vi "TEST - to Line Protocol.vi"() -> ()   [LabVIEW 2020, in "InfluxDB v2 Client.lvlib"]
doc: "Test-VI for \"to Line protocol.vi\""
uses:
  InfluxDB v2 Client.lvlib
  Tag.ctl
  Field.ctl
  Timestamp precision.ctl
  Data Point.ctl
  Data Type.ctl
panel:
  in  "Timestamp precision":T1
  in  "Use Timestamp?":bool
  out "Line Protocol":string
  in  "Data Type":T2
  in  "Field Values":dbl[](array[numeric])=[12.3, 56.7]
  in  "Tags":T3[](array[typedef])=[{"Key"="Host1", "Value"="my_PC"}, {"Key"="Host2", "Value"="X-Server"}]
  in  "Fields":T4[](array[typedef])=[{"Key"="cpu_0", "Value"=variant}, {"Key"="cpu_1", "Value"=variant}]
  in  "Measurement":string="CPU"
  out "Data Point":T5 {"Time Stamp" format="%<%x %.3X>T"}
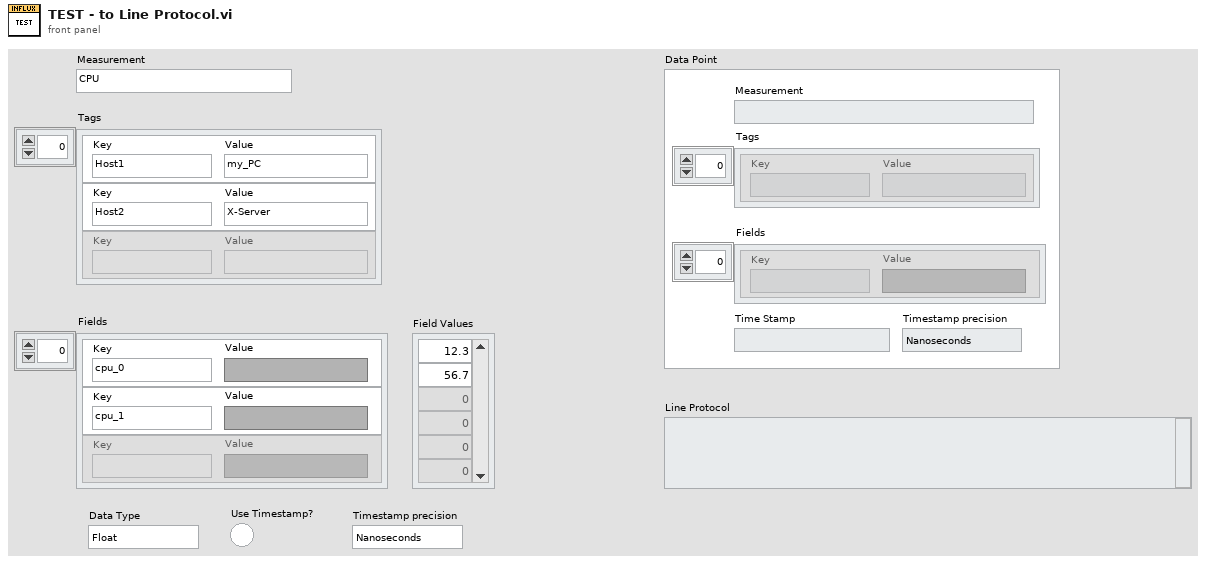
[diagram p1: front panel]
types:
  T1 = typedef "InfluxDB v2 Client.lvlib/Timestamp precision.ctl" = enum16{"Nanoseconds", "Microseconds", "Milliseconds", "Seconds"}
  T2 = typedef "InfluxDB v2 Client.lvlib/Data Type.ctl" = enum16{"Float", "Integer", "UInteger", "String", "Boolean"}
  T3 = typedef "InfluxDB v2 Client.lvlib/Tag.ctl" = cluster{"Key":string, "Value":string}
  T4 = typedef "InfluxDB v2 Client.lvlib/Field.ctl" = cluster{"Key":string, "Value":variant}
  T5 = typedef "InfluxDB v2 Client.lvlib/Data Point.ctl" = cluster{"Measurement":string, "Tags":T3[], "Fields":T4[], "Timestamp precision":T1, "Time Stamp":timestamp}
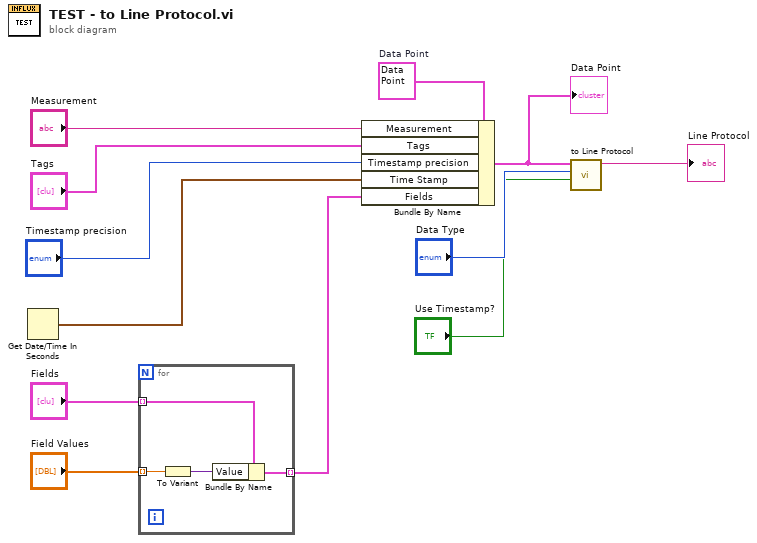
[diagram p0: block diagram]
diagram:
  w12 = T5 {"Measurement"="", "Tags"=[], "Fields"=[], "Timestamp precision"=enum."Nanoseconds", "Time Stamp"=timestamp(0 s since 1904-01-01)}  # Data Point
  n1 = Get Date/Time In Seconds() -> (seconds since 1Jan1904=w1:timestamp)
  n2 = for {
    tunnel: "Fields" -> [w16] mode=indexing
    tunnel: "Field Values" -> [w15] mode=indexing
    tunnel: [w13] -> w3 mode=indexing
    n3 = To Variant(anything=w15) -> (Variant=w14:variant)
    n4 = Bundle By Name(cluster=w16, "Value"=w14) -> (w13:T4)
  }
  n5 = Bundle By Name(cluster=w12, "Measurement"="Measurement", "Tags"="Tags", "Timestamp precision"="Timestamp precision", "Time Stamp"=w1, "Fields"=w3) -> (w9:T5)
  "Data Point" <- w9
  n6 = call "to Line Protocol.vi"(9:"Use Timestamp?", "Use Timestamp?"="Data Type", "Data Point"=w9) -> ("Line Protocol"=→"Line Protocol":string)  [unwired: 7 in, 1 out]
